vi "测试.vi"() -> ()   [LabVIEW 2020]
panel:
  out "Message":string
  out "Done?":bool
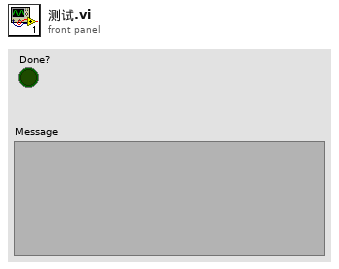
[diagram p1: front panel]
types:
  T1 = cluster{"hSENSOR":i32, "hASIC_T1":i32, "hASIC_T2":i32, "hASIC_P":i32, "hASIC_S":i32}
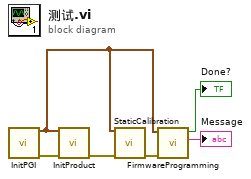
[diagram p0: block diagram]
diagram:
  n1 = call "InitPGI.vi"() -> ("SENSOR"=w4:T1, "error out"=w6:errorcluster)  [unwired: 14 in]
  n2 = call "InitProduct.vi"("SENSOR"=w4, "error in (no error)"=w6) -> ("error out"=w5:errorcluster)  [unwired: 12 in, 1 out]
  n3 = call "StaticCalibration.vi"("SENSOR"=w4, "error in (no error)"=w5) -> ("error out"=w3:errorcluster)  [unwired: 9 in, 4 out]
  n4 = call "FirmwareProgramming.vi"("error in (no error)"=w3, "SENSOR"=w4) -> ("Message"=→"Message":string, "Done?"=→"Done?":bool)  [unwired: 7 in, 1 out]
